vi "Pins Disabled Write.vi"(4 "error in (no error)":errorcluster, 5 "Value":T1(array[ring]), 6 "Container State":T3, 7 "Display State In":T2) -> (0 "error out":errorcluster, 3 "Display State Out":T2)   [LabVIEW 2021, in "roboRIO SPI.xctl"]
uses:
  <vilib>/myRIO/Common/Instrument Driver Framework/Utilities/xctls/roboRIO SPI/roboRIO SPI.xctl
  <vilib>/_xctls/Container State.ctl
  <vilib>/myRIO/Common/Instrument Driver Framework/Utilities/xctls/roboRIO SPI/State.ctl
  <vilib>/myRIO/Common/Instrument Driver Framework/Utilities/xctls/utilities/vis/myRIOXC Error Strings Global.vi
  <vilib>/_xctls/XControlSupport.lvlib
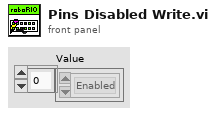
[diagram p1: front panel]
types:
  T1 = enum8{"Enabled", "Disabled", "Disabled and Grayed Out"}[]
  T2 = typedef "roboRIO SPI.xctl/State.ctl" = cluster{"Pin Disabled?":enum8{"Enabled", "Disabled", "Disabled and Grayed Out"}[], "Pin Name":string[]}
  T3 = typedef "XControlSupport.lvlib/Container State.ctl" = cluster{"Indicator?":bool, "Run Mode?":bool, " Refnum":refnum<vi>}
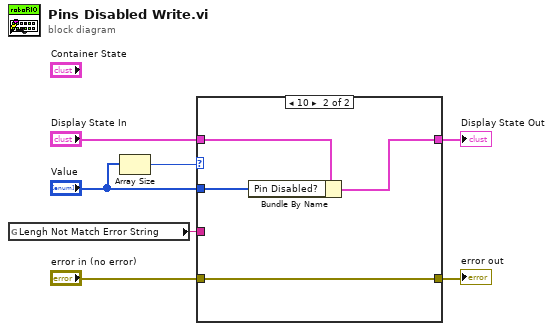
[diagram p0: block diagram]
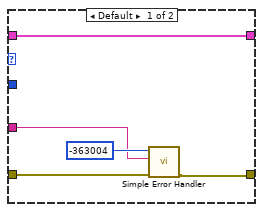
[diagram p2: hidden frame]
diagram:
  n1 = global read "myRIOXC Error Strings Global.vi" "Lengh Not Match Error String"() -> (w1:string)
  n2 = Array Size(array="Value") -> (size(s)=w5:i32)
  n3 = case shown="10" w5 {
    tunnel: "Display State In" -> [w12 w14]
    tunnel: [w12 w16] -> w6
    tunnel: "error in (no error)" -> [w11 w15]
    tunnel: [w10 w15] -> w3
    tunnel: "Value" -> [_ w13]
    tunnel: w1 -> [w8 _]
    frame Default {
      n4 = call <vilib>:"Simple Error Handler.vi"("error code (no error:0)"=-363004, "error source (\" \")"=w8, "error in (no error)"=w11) -> ("error out"=w10:errorcluster)  [unwired: 2 in, 4 out]
    }
    frame 10 {
      n5 = Bundle By Name(cluster=w14, "Pin Disabled?"=w13) -> (w16:T2)
    }
  }
  "error out" <- w3
  "Display State Out" <- w6
